vi "AutoDriveStraight.vi"(8 "error in (no error)":errorcluster, 9 "TimeOut (s)":dbl=99.0, 10 "MaxSpeed (ft/s)":dbl, 11 "Dist (ft)":dbl) -> (0 "error out":errorcluster)   [LabVIEW 2023]
doc: "Wrapper class for drive straight"
uses:
  <vilib>/Utility/semaphor.llb/Obtain Semaphore Reference.vi
  <vilib>/Rock Robotics/WPI/ThirdParty/JAS_Junk/TrajLib/Timer_Reset.vi
  <vilib>/Rock Robotics/WPI/ThirdParty/JAS_Junk/TrajLib/Trajectory_Library.lvlib
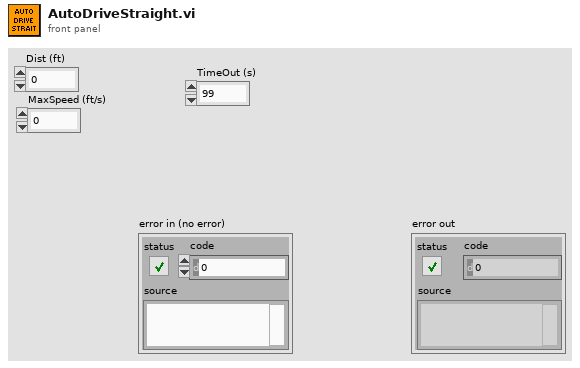
[diagram p1: front panel]
types:
  T1 = typedef "Trajectory_Library.lvlib/TIMER.ctl" = cluster{"StartTime":dbl, "Accumulated TIme":dbl, "Running":bool, "semaphore":T2}
  T2 = typedef "Semaphore RefNum" = refnum<k1>
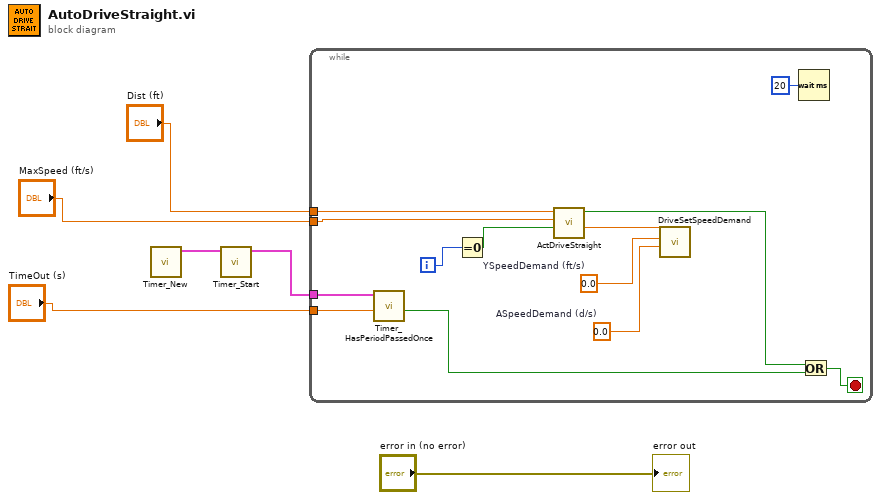
[diagram p0: block diagram]
diagram:
  n1 = call <vilib>:"Timer_New.vi"() -> ("TIMER"=w3:T1)  [unwired: 11 in]
  n2 = call <vilib>:"Timer_Start.vi"("in Timer"=w3) -> ("out Timer"=w2:T1)  [unwired: 10 in]
  n3 = while {
    tunnel: "Dist (ft)" -> [w19]
    tunnel: "MaxSpeed (ft/s)" -> [w18]
    tunnel: w2 -> [w15]
    tunnel: "TimeOut (s)" -> [w14]
    i -> [w16]
    stop <- w12 stop-if-true
    w7 = 0.0  # ASpeedDemand (d/s)
    w8 = 0.0  # YSpeedDemand (ft/s)
    n4 = call <vilib>:"Timer_HasPeriodPassedOnce.vi"("Period"=w14, "in Timer"=w15) -> ("Expired"=w13:bool)  [unwired: 7 in, 2 out]
    n5 = Equal To 0?(x=w16) -> (x = 0?=w17:bool)
    n6 = call "ActDriveStraight.vi"("FirstTime"=w17, "MaxSpeed (ft/s)"=w18, "Dist (ft)"=w19) -> ("XSpeedDemand"=w9:dbl, "Done"=w11:bool)  [unwired: 7 in]
    n7 = call "DriveSetSpeedDemand.vi"("ASpeedDemand (d/s)"=w7, "YSpeedDemand (ft/s)"=w8, "XSpeedDemand (ft/s)"=w9) -> ()  [unwired: 9 in]
    n8 = Wait (ms)(milliseconds to wait=u32 20) -> ()  [unwired: 1 out]
    n9 = Or(x=w11, y=w13) -> (x .or. y?=w12:bool)
  }
  "error out" <- "error in (no error)"
